vi "AFG3352X.reset.vi"(0 "i ref in":refnum<vi>, 3 "ms timeout (10000)":i32=10000, 5 "error in (no error)":errorcluster) -> (14 "i ref out":refnum<vi>, 17 "timed out":bool, 19 "error out":errorcluster)   [LabVIEW 2014, in "AFG3352X.lvlib"]
doc: "Resets the device and enables the output."
uses:
  AFG3352X.lvlib
  CS_Core/CSApplicationBaseClasses/AFGBase/AFGBase.waveformType.ctl
  CSlibraries/UtilityLib/UtilityLib.valueStatus.ctl
  CS_Core/CSApplicationBaseClasses/DeviceBase/DeviceBase.lvlib
  CS_Core/CSApplicationBaseClasses/AFGBase/AFGBase.lvlib
  CSlibraries/UtilityLib/UtilityLib.lvlib
  instr.lib/Agilent 3352X Series/Agilent 3352X Series.lvlib
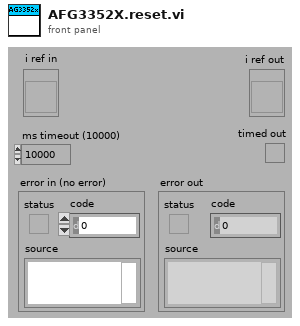
[diagram p1: front panel]
types:
  T1 = typedef "UtilityLib.lvlib/UtilityLib.valueStatus.ctl" = enum16{"no info available", "stand by/off", "on", "warning", "alarm/malfunction", "not implemented", "user action required", "important information", "system default", "control default", "indicator default", "button default"}
  T2 = typedef "AFGBase.lvlib/AFGBase.waveformType.ctl" = enum16{"sine", "square", "ramp", "pulse", "noise", "DC", "arbitrary", "triangle", "ramp_up", "ramp_down", "amplitude modulation"}
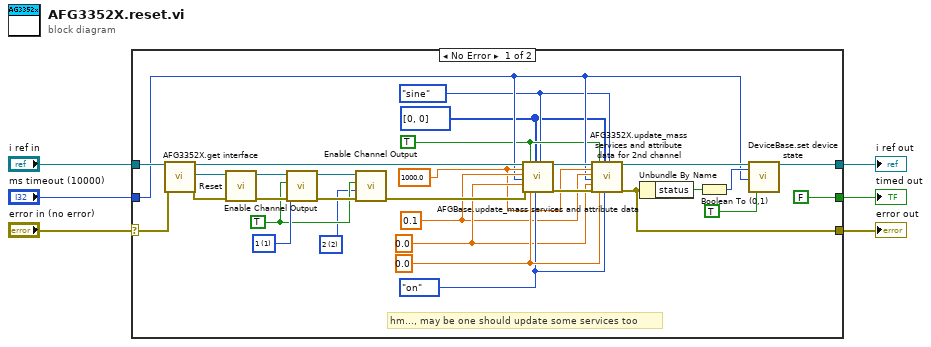
[diagram p0: block diagram]
diagram:
  n1 = case shown="No Error" "error in (no error)" {
    selector: "error in (no error)" -> [w31 w38]
    tunnel: [FALSE _] -> w6
    tunnel: [w35 w39] -> w5
    tunnel: "ms timeout (10000)" -> [w10 _]
    tunnel: "i ref in" -> [w32 w39]
    tunnel: [w18 w38] -> w1
    frame No Error {
      w20 = u16 2 items=["1"=1, "2"=2] ("Channel (1: 1)")
      w25 = u16 1 items=["1"=1, "2"=2] ("Channel (1: 1)")
      w14 = UtilityLib.valueStatus."on" ("valueStatus")
      w15 = 0.0 ("DCOffset")
      w13 = 0.0 ("phase")
      w12 = 0.1 ("amplitude")
      w11 = 1000.0 ("frequency")
      w7 = i16[] [0, 0] ("trigger")
      w8 = AFGBase.waveformType."sine" ("waveformType")
      w9 = TRUE ("enableOutput")
      w21 = TRUE ("Enable Output (T: Enable)")
      # "hm..., may be one should update some services too"
      n2 = call "AFG3352X.get interface.vi"("i ref in"=w32, "error in (no error)"=w31) -> ("i ref out"=w28:refnum<vi>, "interface"=w30:refnum<visa-resource-name>, "error out"=w29:errorcluster)  [unwired: 15 in]
      n3 = call "Reset.vi"("error in (no error)"=w29, "VISA resource name"=w30) -> ("error out"=w26:errorcluster, "VISA resource name out"=w27:refnum<visa-resource-name>)  [unwired: 8 in]
      n4 = call "Enable Channel Output.vi"("error in (no error)"=w26, "Channel (1: 1)"=w25, "Enable Output (T: Enable)"=w21, "VISA resource name"=w27) -> ("error out"=w24:errorcluster, "VISA resource name out"=w22:refnum<visa-resource-name>)  [unwired: 6 in]
      n5 = call "Enable Channel Output.vi"("error in (no error)"=w24, "Channel (1: 1)"=w20, "Enable Output (T: Enable)"=w21, "VISA resource name"=w22) -> ("error out"=w23:errorcluster)  [unwired: 6 in, 1 out]
      n6 = call "AFGBase.update_mass services and attribute data.vi"("i ref in"=w28, "frequency"=w11, "amplitude"=w12, "ms timeout (10000)"=w10, "phase"=w13, "error in (no error)"=w23, "enableOutput"=w9, "DCOffset"=w15, "trigger"=w7, "valueStatus"=w14, "waveformType"=w8) -> ("i ref out"=w17:refnum<vi>, "error out"=w19:errorcluster)  [unwired: 6 in, 1 out]
      n7 = call "AFG3352X.update_mass services and attribute data for 2nd channel.vi"("i ref in"=w17, "frequency"=w11, "amplitude"=w12, "ms timeout (10000)"=w10, "phase"=w13, "error in (no error)"=w19, "enableOutput"=w9, "DCOffset"=w15, "trigger"=w7, "valueStatus"=w14, "waveformType"=w8) -> ("i ref out"=w16:refnum<vi>, "error out"=w18:errorcluster)  [unwired: 6 in, 1 out]
      n8 = Unbundle By Name(w18) -> ("status"=w36:bool)
      n9 = Boolean To (0,1)(Boolean=w36) -> (0, 1=w34:i16)
      n10 = call "DeviceBase.set device state.vi"("i ref in"=w16, "deviceState"=w34, "ms timeout (10000)"=w10, "mayResetError (FALSE)"=TRUE) -> ("i ref out"=w35:refnum<vi>)  [unwired: 13 in, 2 out]
    }
    frame Error {
    }
  }
  "error out" <- w1
  "i ref out" <- w5
  "timed out" <- w6
